vi "main_control_combo_F.vi"(6 "read":bool=TRUE) -> (9 "chiller readout":string, 10 "bytes read":u32)   [LabVIEW 2019]
doc: "The Basic Serial Read and Write example performs a Serial Port Read, a Serial Port Write, or a combination of these actions. The user selects the actions (read or write) on the front panel. If both are selected, the VI will write the data first, read data, and then close the VISA session that is opened to the port. This VI will wait until the specified number of bytes is received at the port. Only the number of bytes specified will be read.\n\nINSTRUCTIONS:\n1) Select the serial resource and configuration parameters (baud rate, data bits, parity, stop bits, flow control).\n2) Select the operations to be performed. \n3) Connect the serial port to your device. If no device is available, perform a loopback test by doing one of the following. Short pins 2 and 3 on a RS-232 cable or short pin 4 to pin 8 and pin 5 to pin 9 on a RS-485/422 cable. \n4) Run the VI to see the data read. (The \"read string\" will match the \"string to write\" if a loopback test was performed.)\n\nNote: The parameters set for the serial port must match the parameters of the connected instrument or device. In this example, the bytes to read parameter specifies the number of bytes that the serial port reads. If there were more bytes at the port than the number specified in bytes to read, those bytes would not be read. Also, if you specify to read more bytes than the number of bytes actually read, you might receive a timeout error message.\n\nOn the block diagram, the Configure Serial Port VI sets the configuration parameters. The front panel displays the controls used to configure the basic parameters, such as baud rate, data bits, and parity. Constants configure the other parameters the user probably does not need set. After the VISA Configure Serial Port VI opens the VISA session and configures the port, the VI passes the VISA resource name to other VIs that perform operations on that VISA resource. The VISA Write function sends a command to the serial device and the VISA Read function returns data based on the command. The VISA Close function then closes the reference to the serial device. It is important to close the reference; otherwise communication through with that port through protocols other than VISA might not be possible."
uses:
  <vilib>/Instr/_visa.llb/VISA Configure Serial Port (Instr).vi
  <vilib>/Utility/file.llb/Read Delimited Spreadsheet (string).vi
  Keithley/Keithley 24XX/Public/Data/Read (Single Point).vi
  Keithley/Keithley 24XX/Keithley 24XX.lvlib
  DELTA ELEKTRONIKA SM Series/DELTA ELEKTRONIKA.lvlib
  <resource>/objmgr/ni.var.rc
panel:
  out "specific error cleared?":bool
  out "manualDelta":bool
  out "read string 7":string
  out "delta readout":string
  in  "delay before read (ms) 4":u32=500
  in  "Combo Box 4":string(combo)
  in  "voltage delta":dbl
  out "delta command":string
  in  "write 4":bool
  in  "stop reading script":bool
  out "bytes read 6":u32
  out "read string 6":string
  out "concatenated string":string
  out "dewpoint":string
  out "temperature":string
  out "humidity":string
  out "n2 flow temperature":string
  out "dewpoint":string
  out "Current Limit 2":bool
  out "Voltage Limit 2":bool
  out "bytes read 5":u32
  out "read string 5":string
  out "bytes read 4":u32
  out "read string 4":string
  out "From Linux Box":string
  in  "Voltage Manual Range (1.0) 2":dbl=1.0
  in  "Current Manual Range (1.0) 2":dbl=1.0
  in  "Resistance Manual Range (1.0) 2":dbl=1.0
  in  "Enable Voltage Auto Range (T:Enable) 2":bool=TRUE
  in  "Enable Current Auto Range (T:Enable) 2":bool=TRUE
  in  "Enable Resistance Auto Range (T:Enable) 2":bool=TRUE
  out "Voltage 3":sgl
  out "Current 3":sgl
  out "Resistance 2":sgl
  out "Current Micro 2":sgl
  out "Command Log and Output":string
  out "COMBO COMMAND":string
  out "all rows":string[][](array[string])
  out "element":i32
  out "current command":string[](array[string])
  out "current argument":string[](array[string])
  out "size(s)":i32
  in  "file path (dialog if empty) 2":path
  in  "Read Script":bool
  in  "Enable Resistance Auto Range (T:Enable)":bool=TRUE
  out "relay TTi":errorcluster
  out "bytes read 3":u32
  out "inverter readout":string
  in  "read 3":bool=TRUE
  in  "delay before read (ms) 3":u32=500
  in  "Combo Box 3":string(combo)="VO?\n"
  in  "voltage or current 2":dbl
  out "string from combo 3":string
  in  "write 3":bool
  out "LV TTi":errorcluster
  out "bytes read 2":u32
  out "LVPS reaout":string
  in  "read 2":bool=TRUE
  in  "delay before read (ms) 2":u32=500
  in  "Combo Box 2":string(combo)="VO?\n"
  in  "voltage or current":dbl
  in  "write 2":bool
  in  "write":bool
  out "string from combo":string
  in  "Temperature":dbl
  in  "Combo Box":string(combo)
  out "Chiller":errorcluster
  out "N2 temperature > dew point + 2C":bool
  in  "File Path of rotonic datalog":path
  out "time humidity temporature dewpoint":string[](array[string])
  in  "Quit":bool
  in  "delay before read (ms)":u32=500
  # "Kiethley Powersupply"
  # "µA"
  # "Delta powersupply Interface"
  # "TTi LV powersupply Interface\nCOM 5 is default"
  # "Medical Chiller Interface\nCOM 6 is default"
  # "TTi LV powersupply Interface for the relay polarity control\nCOM 4 is default"
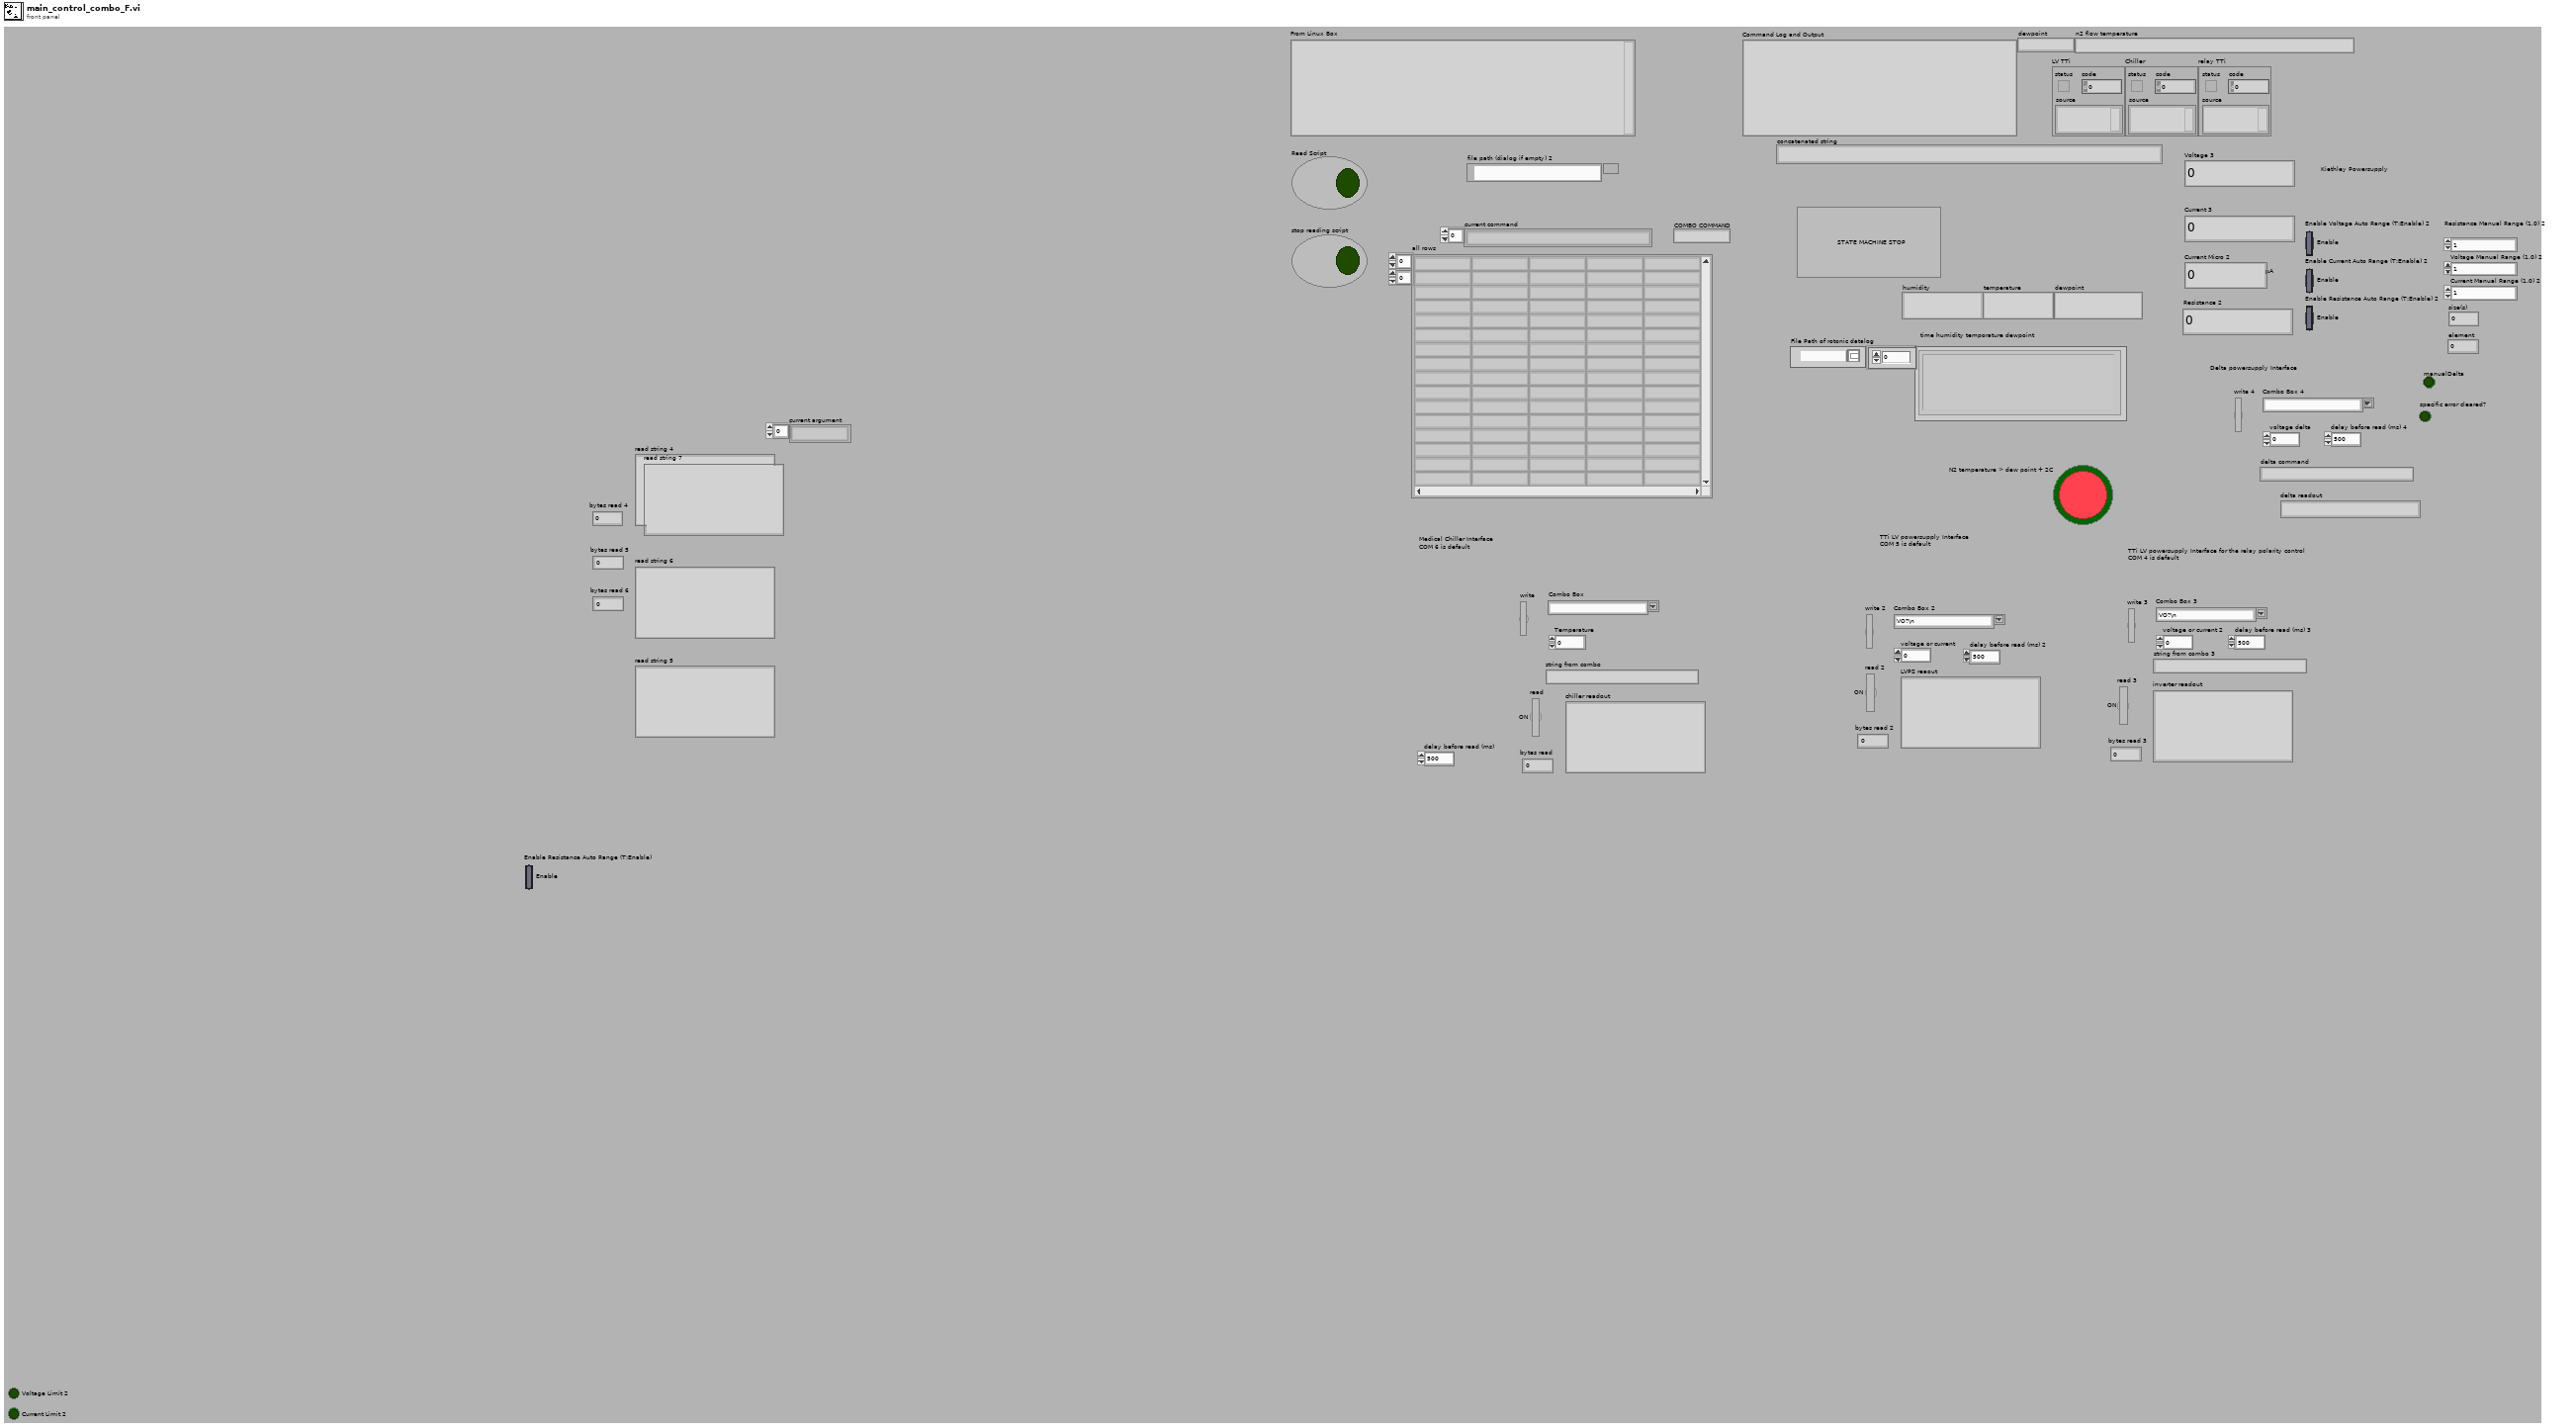
[diagram p1: front panel]
types:
  T1 = cluster{"Baud Rate":u32, "Parity":u16, "Data Bits":u16, "Stop Bits":u16, "Flow Control":u16}
  T2 = enum16{"open", "replace", "create", "open or create", "replace or create", "replace or create with confirmation"}
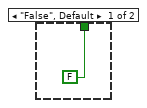
[diagram p2: hidden frame]
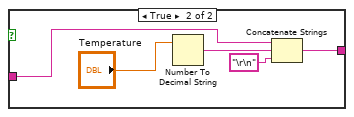
[diagram p4: hidden frame]
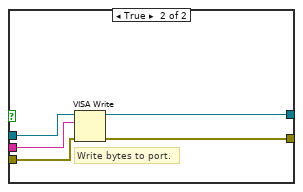
[diagram p5: hidden frame]
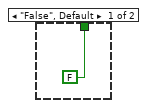
[diagram p7: hidden frame]
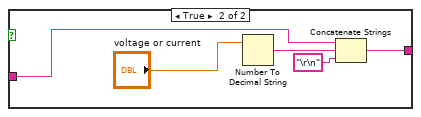
[diagram p9: hidden frame]
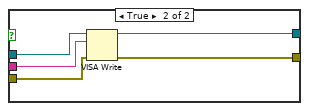
[diagram p10: hidden frame]
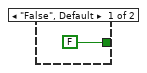
[diagram p12: hidden frame]
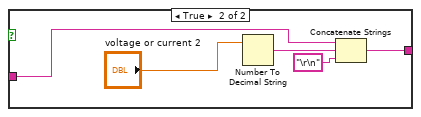
[diagram p14: hidden frame]
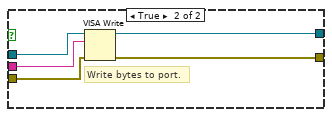
[diagram p15: hidden frame]
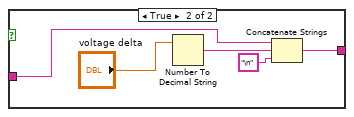
[diagram p18: hidden frame]
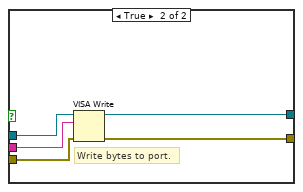
[diagram p19: hidden frame]
diagram:
  # "First save permanent values in non-volatile memory via NI - Max and the *SAV after setting it via SO:VO:MA 52 and SO:CU:MA 30    !"
  n1 = flat-sequence {
    tunnel: [w37] -> w11
    tunnel: [w36] -> w10
    tunnel: [w28] -> w8
    tunnel: [w27] -> w7
    tunnel: [w23] -> w6
    tunnel: [w22] -> w5
    tunnel: [w19] -> w4
    tunnel: [w18] -> w3
    tunnel: [w55] -> w17
    tunnel: [w54] -> w16
    tunnel: [w53] -> w15
    tunnel: [w52] -> w14
    tunnel: [w51] -> w13
    tunnel: w11 -> [w50]
    tunnel: w10 -> [w49]
    tunnel: [w48] -> w9
    tunnel: w8 -> [w47]
    tunnel: w7 -> [w46]
    tunnel: w6 -> [w45]
    tunnel: w5 -> [w44]
    tunnel: w4 -> [w43]
    tunnel: w3 -> [w42]
    tunnel: [w41] -> w2
    tunnel: [w40] -> w1
    tunnel: w17 -> [w661]
    tunnel: w16 -> [w659]
    tunnel: w15 -> [w658]
    tunnel: w14 -> [w656]
    tunnel: w13 -> [w655]
    tunnel: w9 -> [w654]
    tunnel: w2 -> [w653]
    tunnel: w1 -> [w652]
    frame #0 {
      w20 = u32 15000  # timeout (10sec)
      w24 = FALSE  # Enable Termination Char (T)
      w25 = u32 10000  # timeout (10sec)
      w29 = FALSE  # Enable Termination Char (T)
      w30 = u32 10000  # timeout (10sec)
      w35 = u32 10000  # timeout (10sec)
      w33 = FALSE  # Enable Termination Char (T)
      n2 = call "Initialize.vi"("Serial Configuration"=T1 {"Baud Rate"=9600, "Parity"=0, "Data Bits"=8, "Stop Bits"=10, "Flow Control"=1}, "Reset (True)"=FALSE, "VISA resource name"=refnum<visa-resource-name> "COM1" ("VISA resource name 4")) -> ()  [unwired: 7 in, 2 out]
      n3 = call-poly "VISA Configure Serial Port"("VISA resource name"=refnum<visa-resource-name> "COM4", "timeout (10sec)"=w35, "Enable Termination\nChar (T)"=w33) -> ("VISA resource name out"=w36:refnum<visa-resource-name>, "error out"=w37:errorcluster)  [unwired: 11 in]
      n4 = VISA Open(timeout (0)=w20, VISA resource name=refnum<visa-resource-name> "GPIB0::8::INSTR") -> (VISA resource name=w19:refnum<visa-resource-name>, error out=w18:errorcluster)  [unwired: 3 in]
      n5 = call-poly "VISA Configure Serial Port"("VISA resource name"=refnum<visa-resource-name> "COM5", "timeout (10sec)"=w25, "Enable Termination\nChar (T)"=w24) -> ("VISA resource name out"=w22:refnum<visa-resource-name>, "error out"=w23:errorcluster)  [unwired: 11 in]
      n6 = call-poly "VISA Configure Serial Port"("VISA resource name"=refnum<visa-resource-name> "COM6", "timeout (10sec)"=w30, "Enable Termination\nChar (T)"=w29) -> ("VISA resource name out"=w28:refnum<visa-resource-name>, "error out"=w27:errorcluster)  [unwired: 11 in]
    }
    frame #1 {
      # "Disable Output"
      # "State machine for iterating through commands from table"
      n7 = while {
        tunnel: ["Quit"] -> _
        stop <- "Quit" stop-if-true
      }
      n8 = while {
        stop <- w367 stop-if-true
        n9 = local read "Quit"() -> (w367:bool)
        n10 = case shown="True" "Read Script" {
          frame False {
          }
          frame True {
            n11 = Get Date/Time String() -> (date string=w391:string, time string=w389:string)  [unwired: 3 in]
            n12 = Search and Replace String(replace all?=TRUE ("replace all? (F)"), input string=w391, search string="/", replace string="_" ("replace string (\"\")")) -> (result string=w390:string)  [unwired: 4 in, 3 out]
            n13 = Search and Replace String(input string=w389, search string=":", replace string="" ("replace string (\"\")")) -> (result string=w388:string)  [unwired: 5 in, 3 out]
            n14 = Concatenate Strings("C:\\Users\\CMSOTDSF.CERN\\ExecutedCommands\\" ("string"), "command_log_" ("string"), w390, "_" ("string"), w388, ".txt" ("string")) -> (w387:string)
            n15 = String To Path(string=w387) -> (path=w377:path)
            n16 = Open/Create/Replace File(file path (use dialog)=w377, operation (0:open)=T2."replace or create") -> (refnum out=w376:refnum<file>)  [unwired: 4 in, 2 out]
            n17 = Concatenate Strings("Command Log Header for Executed CSV commands " ("text"), "\r\n") -> (w369:string)
            n18 = Set File Position(offset (in bytes) (0)=i64 0, refnum=w376, from (0:start)=enum16{"start", "end", "current"}."end") -> (refnum out=w373:refnum<file>)  [unwired: 1 in, 1 out]
            n19 = Write to Text File(file (use dialog)=w373, text=w369) -> ()  [unwired: 2 in, 3 out]
            n20 = flat-sequence {
              tunnel: ["file path (dialog if empty) 2"] -> w394
              tunnel: [w397] -> w393
              tunnel: [w395] -> w392
              tunnel: w377 -> [w395]
              tunnel: w394 -> [_]
              tunnel: w393 -> [w400]
              tunnel: w392 -> [w399]
              frame #0 {
                # "read table from CSV"
                n21 = call-poly <vilib>:"Read Delimited Spreadsheet.vi"("file path (dialog if empty)"="file path (dialog if empty) 2", "delimiter (\\t)"="," ("delimiter (\\t)")) -> ("all rows"=w397:string[][])  [unwired: 8 in, 5 out]
              }
              frame #1 {
                n22 = Array Size(array=w400) -> (size(s)=w403:i32[])
                n23 = Index Array(array=w403, index #1=0 ("index"), index #2=1 ("index")) -> (element #1=w404:i32)  [unwired: 1 out]
                "element" <- w404
                n24 = for {
                  N: w404 -> [_]
                  tunnel: w400 -> [w421] mode=indexing
                  tunnel: w399 -> [w408]
                  stop <- w414 stop-if-true
                  n25 = local read "Quit"() -> (w416:bool)
                  n26 = Array Subset(array=w421) -> (w417:string[])  [unwired: 2 in]
                  "current command" <- w417
                  n27 = Or(x=w416, y="stop reading script") -> (x .or. y?=w414:bool)
                  n28 = Array Size(array=w417) -> (size(s)=w420:i32)
                  "size(s)" <- w420
                  n29 = Index Array(array=w417, index=0) -> (element=w418:string)
                  "COMBO COMMAND" <- w418
                  n30 = for {
                    N: w420 -> [_]
                    tunnel: w417 -> [w607]
                    i -> [w604]
                    n31 = Add(x=w604, y=1) -> (x+y=w603:i32)
                    n32 = Wait Until Next ms Multiple(millisecond multiple=u32 1000) -> ()  [unwired: 1 out]
                    n33 = Array Subset(array=w607, index=w603) -> (→"current argument":string[])  [unwired: 1 in]
                  }
                  n34 = case shown="\"setChiller\"" w418 {
                    tunnel: w417 -> [w429 w443 w468 w489 w512 w536 _ w550 w571 _]
                    tunnel: [w422 w440 w466 w486 w510 w532 _ _ _ w577] -> w407
                    frame "wait", Default {
                      n35 = Array Subset(array=w429, index=1) -> (w427:string[])  [unwired: 1 in]
                      n36 = Index Array(array=w427, index=0) -> (element=w423:string)
                      n37 = Decimal String To Number(string=w423) -> (number=w425:i32)  [unwired: 2 in, 1 out]
                      n38 = Wait (ms)(milliseconds to wait=w425) -> ()  [unwired: 1 out]
                      n39 = Concatenate Strings("Wait for ", w423) -> (w422:string)
                    }
                    frame "setLVPS" {
                      # "Read the number of bytes specified."
                      # "Write bytes to port."
                      # "MUST specify codes display with single \"\\\""
                      # "Configure Serial port (baud rate,\ndata bits, parity, stop bits and flow control)."
                      n40 = Array Subset(array=w443, index=1) -> (w448:string[])  [unwired: 1 in]
                      n41 = Index Array(array=w448, index #1=0 ("index"), index #2=1 ("index")) -> (element #1=w445:string)  [unwired: 1 out]
                      n42 = Decimal String To Number(string=w445) -> (number=w442:i32)  [unwired: 2 in, 1 out]
                      n43 = To Double Precision Float(number=w442) -> (double precision float=w439:dbl)
                      n44 = case shown="1" w439 {
                        tunnel: ["OP 0\n" ("Combo Box 4") "OP 1\n" ("Combo Box 4")] -> w438
                        frame 0, Default {
                        }
                        frame 1 {
                        }
                      }
                      n45 = VISA Write(VISA resource name=refnum<visa-resource-name> "COM5", write buffer=w438) -> (VISA resource name out=w431:refnum<visa-resource-name>, error out=w430:errorcluster)  [unwired: 1 in, 1 out]
                      n46 = property class="Instr"(reference=w431, error in=w430) -> (reference out=w433:refnum<visa-resource-name>, error out=w434:errorcluster, "Serial Settings:Number of Bytes at Serial Port"=w435:u32)
                      "bytes read 4" <- w435
                      n47 = VISA Read(VISA resource name=w433, byte count=w435, error in (no error)=w434) -> (read buffer=w436:string, error out=w432:errorcluster)  [unwired: 2 out]
                      "read string 4" <- w436
                      n48 = Concatenate Strings("we just set the LV PS voltage to ", w436) -> (w440:string)
                      n49 = call <vilib>:"Simple Error Handler.vi"("error in (no error)"=w432) -> ()  [unwired: 4 in, 5 out]
                    }
                    frame "setDeltaPS" {
                      # "MUST specify codes display with single \"\\\""
                      # "Configure Serial port (baud rate,\ndata bits, parity, stop bits and flow control)."
                      n50 = Array Subset(array=w468, index=1) -> (w472:string[])  [unwired: 1 in]
                      n51 = Index Array(array=w472, index #1=0 ("index"), index #2=1 ("index")) -> (element #1=w459:string)  [unwired: 1 out]
                      n52 = Concatenate Strings("SOUR:VO " ("format string"), w459, "\n" ("string")) -> (w460:string)
                      n53 = VISA Write(VISA resource name=refnum<visa-resource-name> "GPIB0::8::INSTR", write buffer=w460) -> (VISA resource name out=w457:refnum<visa-resource-name>, error out=w456:errorcluster)  [unwired: 1 in, 1 out]
                      n54 = stacked-sequence {
                        tunnel: w456 -> [w475]
                        tunnel: [w475] -> w455
                        tunnel: w457 -> [w474]
                        tunnel: [w474] -> w453
                        frame #0 {
                          n55 = Wait (ms)(milliseconds to wait=u32 500) -> ()  [unwired: 1 out]
                        }
                      }
                      n56 = VISA Write(VISA resource name=w453, write buffer="ME:VO?\n", error in (no error)=w455) -> (VISA resource name out=w451:refnum<visa-resource-name>, error out=w454:errorcluster)  [unwired: 1 out]
                      n57 = VISA Read(VISA resource name=w451, byte count=u32 1024, error in (no error)=w454) -> (read buffer=w464:string, error out=w463:errorcluster)  [unwired: 2 out]
                      "read string 7" <- w464
                      n58 = Concatenate Strings("we just set the Delta voltage to ", w464) -> (w466:string)
                      n59 = call <vilib>:"Simple Error Handler.vi"("error in (no error)"=w463) -> ()  [unwired: 4 in, 5 out]
                    }
                    frame "setInverter" {
                      # "Read the number of bytes specified."
                      # "Write bytes to port."
                      # "MUST specify codes display with single \"\\\""
                      # "Configure Serial port (baud rate,\ndata bits, parity, stop bits and flow control)."
                      n60 = Array Subset(array=w489, index=1) -> (w494:string[])  [unwired: 1 in]
                      n61 = Index Array(array=w494, index #1=0 ("index"), index #2=1 ("index")) -> (element #1=w491:string)  [unwired: 1 out]
                      n62 = Decimal String To Number(string=w491) -> (number=w488:i32)  [unwired: 2 in, 1 out]
                      n63 = To Double Precision Float(number=w488) -> (double precision float=w485:dbl)
                      n64 = case shown="0, Default" w485 {
                        tunnel: ["OP 0\n" ("Combo Box 4") "OP 1\n" ("Combo Box 4")] -> w484
                        frame 0, Default {
                        }
                        frame 1 {
                        }
                      }
                      n65 = VISA Write(VISA resource name=refnum<visa-resource-name> "COM4", write buffer=w484) -> (VISA resource name out=w477:refnum<visa-resource-name>, error out=w476:errorcluster)  [unwired: 1 in, 1 out]
                      n66 = property class="Instr"(reference=w477, error in=w476) -> (reference out=w479:refnum<visa-resource-name>, error out=w480:errorcluster, "Serial Settings:Number of Bytes at Serial Port"=w481:u32)
                      "bytes read 6" <- w481
                      n67 = VISA Read(VISA resource name=w479, byte count=w481, error in (no error)=w480) -> (read buffer=w482:string, error out=w478:errorcluster)  [unwired: 2 out]
                      "read string 6" <- w482
                      n68 = Concatenate Strings("we just set the Inverter voltage to ", w482) -> (w486:string)
                      n69 = call <vilib>:"Simple Error Handler.vi"("error in (no error)"=w478) -> ()  [unwired: 4 in, 5 out]
                    }
                    frame "setChiller" {
                      # "Read the number of bytes specified."
                      # "Write bytes to port."
                      # "MUST specify codes display with single \"\\\""
                      # "Configure Serial port (baud rate,\ndata bits, parity, stop bits and flow control)."
                      n70 = Array Subset(array=w512, index=1) -> (w516:string[])  [unwired: 1 in]
                      n71 = Index Array(array=w516, index #1=0 ("index"), index #2=1 ("index")) -> (element #1=w498:string, element #2=w500:string)
                      n72 = Decimal String To Number(string=w500) -> (number=w499:i32)  [unwired: 2 in, 1 out]
                      n73 = To Double Precision Float(number=w499) -> (double precision float=w497:dbl)
                      n74 = case shown="\"settemp\"" w498 {
                        tunnel: ["STOP\n" ("Combo Box 4") "START\n" ("Combo Box 4") w520] -> w509
                        tunnel: w497 -> [_ _ w519]
                        frame "stop", Default {
                        }
                        frame "start" {
                        }
                        frame "settemp" {
                          n75 = Number To Decimal String(number=w519) -> (decimal integer string=w523:string)  [unwired: 1 in]
                          n76 = Concatenate Strings("OUT_SP_00_" ("Combo Box 4"), w523, "\r\n" ("string")) -> (w520:string)
                        }
                      }
                      n77 = VISA Write(VISA resource name=refnum<visa-resource-name> "COM6", write buffer=w509) -> (VISA resource name out=w502:refnum<visa-resource-name>, error out=w501:errorcluster)  [unwired: 1 in, 1 out]
                      n78 = property class="Instr"(reference=w502, error in=w501) -> (reference out=w504:refnum<visa-resource-name>, error out=w505:errorcluster, "Serial Settings:Number of Bytes at Serial Port"=w506:u32)
                      "bytes read 5" <- w506
                      n79 = VISA Read(VISA resource name=w504, byte count=w506, error in (no error)=w505) -> (read buffer=w507:string, error out=w503:errorcluster)  [unwired: 2 out]
                      "read string 5" <- w507
                      n80 = Concatenate Strings("we just set the Chiller temperature to ", w507) -> (w510:string)
                      n81 = call <vilib>:"Simple Error Handler.vi"("error in (no error)"=w503) -> ()  [unwired: 4 in, 5 out]
                    }
                    frame "keithleynew" {
                      w524 = u16 0 items=["Voltage", "Current"] ("Source Mode  (0: Voltage)")
                      # "Configure each of the three measurements. settings"
                      n82 = Array Subset(array=w536, index=1) -> (w539:string[])  [unwired: 1 in]
                      n83 = Index Array(array=w539, index #1=0 ("index"), index #2=1 ("index")) -> (element #1=w533:string)  [unwired: 1 out]
                      n84 = Decimal String To Number(string=w533) -> (number=w535:i32)  [unwired: 2 in, 1 out]
                      n85 = To Double Precision Float(number=w535) -> (double precision float=w530:dbl)
                      n86 = Concatenate Strings("we just set the keithley voltage to ", w533) -> (w532:string)
                      n87 = call "Configure Output.vi"("Source Mode  (0: Voltage)"=w524, "Compliance  Level (0.1)"=1e-05, "Output Level (0)"=w530, "VISA resource name"=refnum<visa-resource-name> "COM1") -> ("error out"=w528:errorcluster, "VISA resource name out"=w529:refnum<visa-resource-name>)  [unwired: 6 in]
                      n88 = call "Enable Output.vi"("error in (no error)"=w528, "Enable Output (T: Enable)"=TRUE, "VISA resource name"=w529) -> ()  [unwired: 7 in, 2 out]
                    }
                    frame "closekeithley" {
                      n89 = call "Enable Output.vi"("Enable Output (T: Enable)"=FALSE, "VISA resource name"=refnum<visa-resource-name> "COM1") -> ("error out"=w541:errorcluster, "VISA resource name out"=w542:refnum<visa-resource-name>)  [unwired: 8 in]
                      n90 = call "Close.vi"("error in (no error)"=w541, "VISA resource name"=w542) -> ("error out"=w544:errorcluster)  [unwired: 9 in]
                      n91 = call <vilib>:"Simple Error Handler.vi"("error in (no error)"=w544) -> ()  [unwired: 4 in, 5 out]
                    }
                    frame "OldsetDeltaPS" {
                      w565 = TRUE  # Enable Output (T: Enable)
                      # "Read OVP and OCP Status and\nactual voltage and current levels"
                      # "Configure Output"
                      n92 = Array Subset(array=w550, index=1) -> (w555:string[])  [unwired: 1 in]
                      n93 = Index Array(array=w555, index #1=0 ("index"), index #2=1 ("index")) -> (element #1=w552:string, element #2=w547:string)
                      n94 = Decimal String To Number(string=w552) -> (number=w549:i32)  [unwired: 2 in, 1 out]
                      n95 = Decimal String To Number(string=w547) -> (number=w548:i32)  [unwired: 2 in, 1 out]
                      n96 = To Double Precision Float(number=w549) -> (double precision float=w545:dbl)
                      n97 = To Double Precision Float(number=w548) -> (double precision float=w546:dbl)
                      n98 = call "Configure Output Voltage.vi"("Set Voltage(0.0 V)"=w545, "VISA resource name"=refnum<visa-resource-name> "LPT1") -> ("error out"=w564:errorcluster, "VISA resource name out"=w563:refnum<visa-resource-name>)  [unwired: 8 in]
                      n99 = call "Configure Current Limit.vi"("error in (no error)"=w564, "Current Limit (0.0 A)"=w546, "VISA resource name"=w563) -> ("error out"=w566:errorcluster, "VISA resource name out"=w567:refnum<visa-resource-name>)  [unwired: 7 in]
                      n100 = call "Configure Output.vi"("Enable Output (T: Enable)"=w565, "error in (no error)"=w566, "VISA resource name"=w567) -> ("error out"=w557:errorcluster, "VISA resource name out"=w556:refnum<visa-resource-name>)  [unwired: 7 in]
                      n101 = call "Output Protection Status.vi"("error in (no error)"=w557, "VISA resource name"=w556) -> ("error out"=w559:errorcluster, "OCP Tripped?"=→"Current Limit 2":bool, "OVP Tripped?"=→"Voltage Limit 2":bool, "VISA resource name out"=w558:refnum<visa-resource-name>)  [unwired: 6 in]
                      n102 = call "Read Output.vi"("error in (no error)"=w559, "VISA resource name"=w558) -> ()  [unwired: 6 in, 4 out]
                    }
                    frame "dumsetDeltaPS" {
                      n103 = Array Subset(array=w571, index=1) -> (w576:string[])  [unwired: 1 in]
                      n104 = Index Array(array=w576, index #1=0 ("index"), index #2=1 ("index")) -> (element #1=w573:string, element #2=w568:string)
                      n105 = Decimal String To Number(string=w573) -> (number=w570:i32)  [unwired: 2 in, 1 out]
                      n106 = Decimal String To Number(string=w568) -> (number=w569:i32)  [unwired: 2 in, 1 out]
                      n107 = To Double Precision Float(number=w570) -> ()  [unwired: 1 out]
                      n108 = To Double Precision Float(number=w569) -> ()  [unwired: 1 out]
                    }
                    frame "2sCalibration" {
                      # "C:\\Users\\CMSOTDSF.CERN\\2sCalibrationOut"
                      # "run a windows batch file that will call ssh command with an INPUT bash script\nThe input bash script will run the 2s calibration and is located here:\nC:\\Users\\CMSOTDSF.CERN\\cc7.sh"
                      n109 = flat-sequence {
                        tunnel: [w580] -> w578
                        tunnel: w578 -> [w586]
                        tunnel: [w585] -> w577
                        frame #0 {
                          n110 = call <vilib>:"System Exec.vi"("run minimized? (F)"=TRUE, "working directory"=path "C:/Users/CMSOTDSF.CERN/OpenSSH", "command line"="cmd /c C:\\Users\\CMSOTDSF.CERN\\windows_cc7.bat") -> ("standard error"=w581:string, "standard output"=w582:string)  [unwired: 5 in, 2 out]
                          "From Linux Box" <- w582
                          n111 = Concatenate Strings(w582, w581) -> (w580:string)
                        }
                        frame #1 {
                          n112 = Get Date/Time String() -> (date string=w597:string, time string=w599:string)  [unwired: 3 in]
                          n113 = Search and Replace String(input string=w599, search string=":", replace string="" ("replace string (\"\")")) -> (result string=w600:string)  [unwired: 5 in, 3 out]
                          n114 = Search and Replace String(replace all?=TRUE ("replace all? (F)"), input string=w597, search string="/", replace string="_" ("replace string (\"\")")) -> (result string=w598:string)  [unwired: 4 in, 3 out]
                          n115 = Concatenate Strings("C:\\Users\\CMSOTDSF.CERN\\2sCalibrationOut\\" ("string"), "2scalibration_" ("string"), w598, "_" ("string"), w600, ".txt" ("string")) -> (w601:string)
                          n116 = String To Path(string=w601) -> (path=w602:path)
                          n117 = Concatenate Strings("2S Calibration done output is saved to: ", w601) -> (w585:string)
                          n118 = Write to Text File(file (use dialog)=w602, text=w586) -> ()  [unwired: 2 in, 3 out]
                        }
                      }
                    }
                  }
                  "Command Log and Output" <- w407
                  n119 = Open/Create/Replace File(file path (use dialog)=w408, operation (0:open)=T2."open") -> (refnum out=w409:refnum<file>)  [unwired: 4 in, 2 out]
                  n120 = Concatenate Strings(w407, "\r\n") -> (w406:string)
                  n121 = Set File Position(offset (in bytes) (0)=i64 0, refnum=w409, from (0:start)=enum16{"start", "end", "current"}."end") -> (refnum out=w411:refnum<file>)  [unwired: 1 in, 1 out]
                  n122 = Write to Text File(file (use dialog)=w411, text=w406) -> ()  [unwired: 2 in, 3 out]
                }
                "all rows" <- w400
              }
              frame #2 {
                n123 = invoke on="Read Script" class="Bool (strict)" method="Reinit To Default"() -> ()  [unwired: 3 in, 3 out]
                n124 = local write "COMBO COMMAND"("" ("COMBO COMMAND")) -> ()
              }
            }
          }
        }
      }
      n125 = while {
        tunnel: w43 -> [w266]
        tunnel: [w260] -> w41
        tunnel: w42 -> [w265]
        tunnel: [w259] -> w40
        stop <- w261 stop-if-true
        n126 = local read "COMBO COMMAND"() -> (w256:string)
        n127 = Search and Replace String(input string=w256, search string="setDeltaPS", replace string="True" ("replace string (\"\")")) -> (result string=w262:string)  [unwired: 5 in, 3 out]
        n128 = case shown="\"False\", Default" w262 {
          tunnel: [FALSE TRUE] -> w263
          frame "False", Default {
          }
          frame "True" {
          }
        }
        n129 = local read "Quit"() -> (w264:bool)
        n130 = Or(x=w263, y=w264) -> (x .or. y?=w258:bool)
        n131 = Not(x=w258) -> (.not. x?=w257:bool)
        "manualDelta" <- w257
        n132 = case shown="True" w257 {
          tunnel: w266 -> [w268 w272]
          tunnel: w265 -> [w267 w271]
          tunnel: [w268 w270] -> w260
          tunnel: [w267 w269] -> w259
          frame False {
          }
          frame True {
            n133 = while {
              tunnel: w272 -> [w292]
              tunnel: [w278] -> w270
              tunnel: w271 -> [w275]
              tunnel: [w277] -> w269
              stop <- FALSE stop-if-true
              # "delta"
              # "Configure Serial port (baud rate,\ndata bits, parity, stop bits and flow control)."
              n134 = call <vilib>:"Clear Errors.vi"("error in (no error)"=w275, "specific error code to clear (0: all)"=-1073807339.0 ("y")) -> ("error out"=w274:errorcluster, "specific error cleared?"=→"specific error cleared?":bool)  [unwired: 4 in]
              n135 = Match True/False String(2:"" ("false string"), 3:"SOUR:VO " ("format string"), 4:"Combo Box 4") -> (0:w285:bool)  [unwired: 1 out]
              n136 = case shown="False" w285 {
                tunnel: [w293 w296] -> w282
                tunnel: "Combo Box 4" -> [w293 w295]
                frame False {
                }
                frame True {
                  n137 = Number To Decimal String(number="voltage delta") -> (decimal integer string=w298:string)  [unwired: 1 in]
                  n138 = Concatenate Strings(w295, w298, "\n" ("string")) -> (w296:string)
                }
              }
              "delta command" <- w282
              n139 = case shown="False" "write 4" {
                tunnel: [w302 w311] -> w291
                tunnel: w292 -> [w306 w310]
                tunnel: w274 -> [w305 w309]
                tunnel: [w303 w308] -> w289
                tunnel: w282 -> [_ w307]
                frame False {
                  n140 = VISA Write(VISA resource name=w306, write buffer="ME:VO?\n", error in (no error)=w305) -> (VISA resource name out=w303:refnum<visa-resource-name>, error out=w302:errorcluster)  [unwired: 1 out]
                }
                frame True {
                  # "Write bytes to port."
                  n141 = VISA Write(VISA resource name=w310, write buffer=w307, error in (no error)=w309) -> (VISA resource name out=w308:refnum<visa-resource-name>, error out=w311:errorcluster)  [unwired: 1 out]
                }
              }
              n142 = stacked-sequence {
                tunnel: w291 -> [w301]
                tunnel: [w301] -> w290
                tunnel: w289 -> [w300]
                tunnel: [w300] -> w288
                frame #0 {
                  n143 = Wait (ms)(milliseconds to wait="delay before read (ms) 4") -> ()  [unwired: 1 out]
                }
              }
              n144 = Not(x="write 4") -> (.not. x?=w280:bool)
              n145 = case shown="True" w280 {
                tunnel: w290 -> [w313 w314]
                tunnel: [w313 w319] -> w277
                tunnel: [w312 w318] -> w278
                tunnel: w288 -> [w312 w316]
                frame False {
                }
                frame True {
                  # "Read the number of bytes specified."
                  n146 = VISA Read(VISA resource name=w316, byte count=u32 1024, error in (no error)=w314) -> (VISA resource name out=w318:refnum<visa-resource-name>, read buffer=→"delta readout":string, error out=w319:errorcluster)  [unwired: 1 out]
                }
              }
              n147 = Wait Until Next ms Multiple(millisecond multiple=u32 50) -> ()  [unwired: 1 out]
            }
          }
        }
        n148 = local read "Quit"() -> (w261:bool)
      }
      n149 = while {
        tunnel: w44 -> [w132]
        tunnel: [w134] -> w51
        tunnel: w45 -> [w133]
        tunnel: [w135] -> w52
        stop <- w131 stop-if-true
        n150 = local read "COMBO COMMAND"() -> (w127:string)
        n151 = Search and Replace String(input string=w127, search string="setLVPS", replace string="True" ("replace string (\"\")")) -> (result string=w128:string)  [unwired: 5 in, 3 out]
        n152 = case shown="\"True\"" w128 {
          tunnel: [FALSE TRUE] -> w129
          frame "False", Default {
          }
          frame "True" {
          }
        }
        n153 = local read "Quit"() -> (w130:bool)
        n154 = Or(x=w129, y=w130) -> (x .or. y?=w124:bool)
        n155 = Not(x=w124) -> (.not. x?=w123:bool)
        n156 = case shown="True" w123 {
          tunnel: [w138 w143] -> w135
          tunnel: [w139 w142] -> w134
          tunnel: w133 -> [w138 w141]
          tunnel: w132 -> [w139 w140]
          frame False {
          }
          frame True {
            n157 = while {
              shift-right: [w157] -> w143
              shift-left: w141 -> [w159]
              shift-right: [w156] -> w142
              shift-left: w140 -> [w158]
              stop <- FALSE stop-if-true
              # "TTi SEH PS LV"
              n158 = Match True/False String(2:"" ("false string"), 3:"OUT_SP_00_" ("format string"), 4:"Combo Box 2") -> (0:w149:bool)  [unwired: 1 out]
              n159 = case shown="False" w149 {
                tunnel: [w161 w164] -> w146
                tunnel: "Combo Box 2" -> [w161 w163]
                frame False {
                }
                frame True {
                  n160 = Number To Decimal String(number="voltage or current") -> (decimal integer string=w166:string)  [unwired: 1 in]
                  n161 = Concatenate Strings(w163, w166, "\r\n" ("string")) -> (w164:string)
                }
              }
              n162 = case shown="False" "write 2" {
                tunnel: [w171 w176] -> w155
                tunnel: w158 -> [w170 w175]
                tunnel: w159 -> [w171 w174]
                tunnel: [w170 w173] -> w153
                tunnel: w146 -> [_ w172]
                frame False {
                }
                frame True {
                  n163 = VISA Write(VISA resource name=w175, write buffer=w172, error in (no error)=w174) -> (VISA resource name out=w173:refnum<visa-resource-name>, error out=w176:errorcluster)  [unwired: 1 out]
                }
              }
              n164 = stacked-sequence {
                tunnel: w155 -> [w169]
                tunnel: [w169] -> w154
                tunnel: w153 -> [w168]
                tunnel: [w168] -> w152
                frame #0 {
                  n165 = Wait (ms)(milliseconds to wait="delay before read (ms) 2") -> ()  [unwired: 1 out]
                }
              }
              n166 = case shown="True" "read 2" {
                tunnel: w154 -> [w178 w182]
                tunnel: [w178 w186] -> w157
                tunnel: [w177 w185] -> w156
                tunnel: w152 -> [w177 w184]
                frame False {
                }
                frame True {
                  # "Read the number of bytes specified."
                  n167 = property class="Instr"(reference=w184, error in=w182) -> (reference out=w183:refnum<visa-resource-name>, error out=w181:errorcluster, "Serial Settings:Number of Bytes at Serial Port"=w180:u32)
                  "bytes read 2" <- w180
                  n168 = VISA Read(VISA resource name=w183, byte count=w180, error in (no error)=w181) -> (VISA resource name out=w185:refnum<visa-resource-name>, read buffer=→"LVPS reaout":string, error out=w186:errorcluster)  [unwired: 1 out]
                }
              }
              n169 = Wait Until Next ms Multiple(millisecond multiple=u32 50) -> ()  [unwired: 1 out]
            }
          }
        }
        n170 = local read "Quit"() -> (w131:bool)
      }
      n171 = while {
        tunnel: w50 -> [w197]
        tunnel: [w199] -> w54
        tunnel: w49 -> [w196]
        tunnel: [w198] -> w53
        stop <- w195 stop-if-true
        n172 = local read "COMBO COMMAND"() -> (w194:string)
        n173 = Search and Replace String(input string=w194, search string="setInverter", replace string="True" ("replace string (\"\")")) -> (result string=w193:string)  [unwired: 5 in, 3 out]
        n174 = case shown="\"True\"" w193 {
          tunnel: [FALSE TRUE] -> w190
          frame "False", Default {
          }
          frame "True" {
          }
        }
        n175 = local read "Quit"() -> (w189:bool)
        n176 = Or(x=w190, y=w189) -> (x .or. y?=w188:bool)
        n177 = Not(x=w188) -> (.not. x?=w187:bool)
        n178 = case shown="True" w187 {
          tunnel: [w203 w207] -> w199
          tunnel: [w202 w206] -> w198
          tunnel: w197 -> [w203 w205]
          tunnel: w196 -> [w202 w204]
          frame False {
          }
          frame True {
            n179 = while {
              shift-right: [w222] -> w207
              shift-left: w205 -> [w223]
              shift-right: [w221] -> w206
              shift-left: w204 -> [w209]
              stop <- FALSE stop-if-true
              # "RELAY LV PS"
              # "Configure Serial port (baud rate,\ndata bits, parity, stop bits and flow control)."
              n180 = Match True/False String(2:"" ("false string"), 3:"OUT_SP_00_" ("format string"), 4:"Combo Box 3") -> (0:w214:bool)  [unwired: 1 out]
              n181 = case shown="False" w214 {
                tunnel: [w225 w228] -> w211
                tunnel: "Combo Box 3" -> [w225 w227]
                frame False {
                }
                frame True {
                  n182 = Number To Decimal String(number="voltage or current 2") -> (decimal integer string=w230:string)  [unwired: 1 in]
                  n183 = Concatenate Strings(w227, w230, "\r\n" ("string")) -> (w228:string)
                }
              }
              "string from combo 3" <- w211
              n184 = case shown="False" "write 3" {
                tunnel: [w235 w243] -> w220
                tunnel: w209 -> [w238 w242]
                tunnel: w223 -> [w234 w241]
                tunnel: [w236 w240] -> w218
                tunnel: w211 -> [_ w239]
                frame False {
                  n185 = VISA Write(VISA resource name=w238, write buffer="VO?\n", error in (no error)=w234) -> (VISA resource name out=w236:refnum<visa-resource-name>, error out=w235:errorcluster)  [unwired: 1 out]
                }
                frame True {
                  # "Write bytes to port."
                  n186 = VISA Write(VISA resource name=w242, write buffer=w239, error in (no error)=w241) -> (VISA resource name out=w240:refnum<visa-resource-name>, error out=w243:errorcluster)  [unwired: 1 out]
                }
              }
              n187 = stacked-sequence {
                tunnel: w220 -> [w233]
                tunnel: [w233] -> w219
                tunnel: w218 -> [w232]
                tunnel: [w232] -> w217
                frame #0 {
                  n188 = Wait (ms)(milliseconds to wait="delay before read (ms) 3") -> ()  [unwired: 1 out]
                }
              }
              n189 = case shown="True" "read 3" {
                tunnel: w219 -> [w245 w249]
                tunnel: [w245 w253] -> w222
                tunnel: [w244 w252] -> w221
                tunnel: w217 -> [w244 w251]
                frame False {
                }
                frame True {
                  # "Read the number of bytes specified."
                  n190 = property class="Instr"(reference=w251, error in=w249) -> (reference out=w250:refnum<visa-resource-name>, error out=w248:errorcluster, "Serial Settings:Number of Bytes at Serial Port"=w247:u32)
                  "bytes read 3" <- w247
                  n191 = VISA Read(VISA resource name=w250, byte count=w247, error in (no error)=w248) -> (VISA resource name out=w252:refnum<visa-resource-name>, read buffer=→"inverter readout":string, error out=w253:errorcluster)  [unwired: 1 out]
                }
              }
              n192 = Wait Until Next ms Multiple(millisecond multiple=u32 50) -> ()  [unwired: 1 out]
            }
          }
        }
        n193 = local read "Quit"() -> (w195:bool)
      }
      n194 = while {
        tunnel: w47 -> [w66]
        tunnel: [w67] -> w48
        tunnel: w46 -> [w65]
        tunnel: [w68] -> w55
        stop <- w64 stop-if-true
        n195 = local read "COMBO COMMAND"() -> (w62:string)
        n196 = Search and Replace String(input string=w62, search string="setChiller", replace string="True" ("replace string (\"\")")) -> (result string=w60:string)  [unwired: 5 in, 3 out]
        n197 = case shown="\"True\"" w60 {
          tunnel: [FALSE TRUE] -> w61
          frame "False", Default {
          }
          frame "True" {
          }
        }
        n198 = local read "Quit"() -> (w63:bool)
        n199 = Or(x=w61, y=w63) -> (x .or. y?=w57:bool)
        n200 = Not(x=w57) -> (.not. x?=w56:bool)
        n201 = case shown="True" w56 {
          tunnel: [w71 w76] -> w68
          tunnel: [w72 w75] -> w67
          tunnel: w66 -> [w72 w74]
          tunnel: w65 -> [w71 w73]
          frame False {
          }
          frame True {
            n202 = while {
              shift-right: [w90] -> w76
              shift-left: w73 -> [w92]
              shift-right: [w89] -> w75
              shift-left: w74 -> [w91]
              stop <- FALSE stop-if-true
              # "CHILLER"
              # "Configure Serial port (baud rate,\ndata bits, parity, stop bits and flow control)."
              n203 = Match True/False String(2:"" ("false string"), 3:"OUT_SP_00_" ("format string"), 4:"Combo Box") -> (0:w82:bool)  [unwired: 1 out]
              n204 = case shown="False" w82 {
                tunnel: [w94 w97] -> w79
                tunnel: "Combo Box" -> [w94 w96]
                frame False {
                }
                frame True {
                  n205 = Number To Decimal String(number="Temperature") -> (decimal integer string=w99:string)  [unwired: 1 in]
                  n206 = Concatenate Strings(w96, w99, "\r\n" ("string")) -> (w97:string)
                }
              }
              "string from combo" <- w79
              n207 = case shown="False" "write" {
                tunnel: [w103 w112] -> w88
                tunnel: w91 -> [w107 w111]
                tunnel: w92 -> [w106 w110]
                tunnel: [w104 w109] -> w86
                tunnel: w79 -> [_ w108]
                frame False {
                  n208 = VISA Write(VISA resource name=w107, write buffer="IN_PV_00\r\n", error in (no error)=w106) -> (VISA resource name out=w104:refnum<visa-resource-name>, error out=w103:errorcluster)  [unwired: 1 out]
                }
                frame True {
                  # "Write bytes to port."
                  n209 = VISA Write(VISA resource name=w111, write buffer=w108, error in (no error)=w110) -> (VISA resource name out=w109:refnum<visa-resource-name>, error out=w112:errorcluster)  [unwired: 1 out]
                }
              }
              n210 = stacked-sequence {
                tunnel: w88 -> [w102]
                tunnel: [w102] -> w87
                tunnel: w86 -> [w101]
                tunnel: [w101] -> w85
                frame #0 {
                  n211 = Wait (ms)(milliseconds to wait="delay before read (ms)") -> ()  [unwired: 1 out]
                }
              }
              n212 = case shown="True" "read" {
                tunnel: w87 -> [w114 w118]
                tunnel: [w114 w122] -> w90
                tunnel: [w113 w121] -> w89
                tunnel: w85 -> [w113 w120]
                frame False {
                }
                frame True {
                  # "Read the number of bytes specified."
                  n213 = property class="Instr"(reference=w120, error in=w118) -> (reference out=w119:refnum<visa-resource-name>, error out=w117:errorcluster, "Serial Settings:Number of Bytes at Serial Port"=w116:u32)
                  "bytes read" <- w116
                  n214 = VISA Read(VISA resource name=w119, byte count=w116, error in (no error)=w117) -> (VISA resource name out=w121:refnum<visa-resource-name>, read buffer=→"chiller readout":string, error out=w122:errorcluster)  [unwired: 1 out]
                }
              }
              n215 = Wait Until Next ms Multiple(millisecond multiple=u32 50) -> ()  [unwired: 1 out]
            }
          }
        }
        n216 = local read "Quit"() -> (w64:bool)
      }
      n217 = while {
        stop <- w610 stop-if-true
        (unwired) "humidity_202105"
        (unwired) path "C:/Users/fengwang.PCCMSTKUPDSF2/Desktop/RotronicUSBDriver/dataLog" ("file (use dialog)")
        # "dew point"
        # "N2 flow temperature"
        # "Convert text file string to array"
        # "Return the Number of lines."
        # "Extract only the size dimension we need"
        # "Get the size of the array"
        # "Read Text File, dialog box if none"
        n218 = local read "Quit"() -> (w610:bool)
        n219 = Get Date/Time In Seconds() -> (seconds since 1Jan1904=w616:timestamp)
        n220 = Format Date/Time String(time format string (%c)="%d_%m_%Y", seconds (now)=w616) -> (date/time string=w614:string)  [unwired: 1 in]
        n221 = Concatenate Strings("C:\\Users\\fengwang.PCCMSTKUPDSF2\\Desktop\\RotronicUSBDriver\\dataLog\\humidity_", w614) -> (→"concatenated string":string)
        n222 = Read from Text File(file (use dialog)="File Path of rotonic datalog") -> (text=w643:string)  [unwired: 1 in, 5 out]
        n223 = Spreadsheet String To Array(delimiter (Tab)="\r", format string="%d", spreadsheet string=w643) -> (array=w641:dbl[][])  [unwired: 1 out]
        n224 = Array Size(array=w641) -> (size(s)=w642:i32[])
        n225 = Index Array(array=w642) -> (element=w645:i32)  [unwired: 1 in]
        n226 = Read from Text File(file (use dialog)="File Path of rotonic datalog", count=w645) -> (text=w646:string[])  [unwired: 1 in, 4 out]
        n227 = Decrement(x=w645) -> (x-1=w644:i32)
        n228 = Array Subset(array=w646, index=w644) -> (w647:string[])  [unwired: 1 in]
        "time humidity temporature dewpoint" <- w647
        n229 = Get Date/Time In Seconds() -> (seconds since 1Jan1904=w639:timestamp)
        n230 = Array To Spreadsheet String(array=w647, 3:"%d/%m/%Y %H:%M:%S %4.12f %4.12f %4.12f" ("time format string (%c)")) -> (spreadsheet string=w618:string)  [unwired: 1 in]
        n231 = Format Date/Time String(time format string (%c)="%d/%m/%Y %H:%M:%S ", seconds (now)=w639) -> (date/time string=w640:string)  [unwired: 1 in]
        n232 = String Subset(string=w618, offset (0)=20, length (rest)=5 ("length (rest)")) -> (substring=→"humidity":string)
        n233 = Scan From String(format string=w640, input string=w618) -> (remaining string=w648:string)  [unwired: 4 in, 2 out]
        n234 = String Subset(string=w618, offset (0)=27, length (rest)=5 ("length (rest)")) -> (substring=→"temperature":string)
        n235 = String Subset(string=w618, offset (0)=34, length (rest)=6 ("length (rest)")) -> (substring=w611:string)
        "dewpoint" <- w611
        n236 = property class="Variable Object" props=["ClassId"](reference=w611) -> ()  [unwired: 1 in, 3 out]
        n237 = String Subset(string=w648, offset (0)=12, length (rest)=5 ("length (rest)")) -> (substring=w649:string)
        "dewpoint" <- w649
        n238 = Fract/Exp String To Number(string=w649) -> (number=w629:dbl)  [unwired: 3 in, 1 out]
        n239 = String Subset(string=w648, offset (0)=6, length (rest)=5 ("length (rest)")) -> (substring=w627:string)
        "n2 flow temperature" <- w627
        n240 = Fract/Exp String To Number(string=w627) -> (number=w650:dbl)  [unwired: 3 in, 1 out]
        n241 = Add(x=w629, y=2.0) -> (x+y=w628:dbl)
        n242 = Greater?(x=w650, y=w628) -> (0:→"N2 temperature > dew point + 2C":bool)
        n243 = call <vilib>:"Simple Error Handler.vi"() -> ()  [unwired: 5 in, 5 out]
      }
      n244 = while {
        stop <- w323 stop-if-true
        n245 = local read "file path (dialog if empty) 2"() -> (w324:path)
        n246 = Equal?(x=w324, y=path "") -> (x = y?=w328:bool)
        n247 = case shown="False" w328 {
          tunnel: [w330 path "C:/LabVIEW/OuterTrackerControl/example_commands.csv"] -> w329
          tunnel: w324 -> [w330 _]
          frame False {
          }
          frame True {
          }
        }
        n248 = local read "Quit"() -> (w323:bool)
        n249 = call-poly <vilib>:"Read Delimited Spreadsheet.vi"("file path (dialog if empty)"=w329, "delimiter (\\t)"="," ("delimiter (\\t)")) -> ("all rows"=w327:string[][])  [unwired: 8 in, 5 out]
        n250 = local write "all rows"(w327) -> ()
      }
      n251 = while {
        stop <- w334 stop-if-true
        w350 = u16 0 items=["Volts", "Current", "Resistance"]  # Function (0: Volts)
        w357 = u16 2 items=["Volts", "Current", "Resistance"]  # Function (0: Volts)
        w358 = u16 1 items=["Volts", "Current", "Resistance"]  # Function (0: Volts)
        # "Take the readings."
        # "Configure the output."
        # "Configure each of the three measurements. settings"
        n252 = call "Configure Measurement.vi"("Manual Range (1.0)"="Voltage Manual Range (1.0) 2", "Enable Auto Range (T:Enable)"="Enable Voltage Auto Range (T:Enable) 2", "Function (0: Volts)"=w350, "VISA resource name"=refnum<visa-resource-name> "COM1") -> ("error out"=w361:errorcluster, "VISA resource name out"=w362:refnum<visa-resource-name>)  [unwired: 6 in]
        n253 = call "Configure Measurement.vi"("Manual Range (1.0)"="Current Manual Range (1.0) 2", "error in (no error)"=w361, "Enable Auto Range (T:Enable)"="Enable Current Auto Range (T:Enable) 2", "Function (0: Volts)"=w358, "VISA resource name"=w362) -> ("error out"=w360:errorcluster, "VISA resource name out"=w359:refnum<visa-resource-name>)  [unwired: 5 in]
        n254 = call "Configure Measurement.vi"("Manual Range (1.0)"="Resistance Manual Range (1.0) 2", "error in (no error)"=w360, "Enable Auto Range (T:Enable)"="Enable Resistance Auto Range (T:Enable) 2", "Function (0: Volts)"=w357, "VISA resource name"=w359) -> ("error out"=w339:errorcluster, "VISA resource name out"=w340:refnum<visa-resource-name>)  [unwired: 5 in]
        n255 = local read "COMBO COMMAND"() -> (w338:string)
        n256 = call "Enable Output.vi"("error in (no error)"=w339, "Enable Output (T: Enable)"=TRUE, "VISA resource name"=w340) -> ("error out"=w343:errorcluster, "VISA resource name out"=w342:refnum<visa-resource-name>)  [unwired: 7 in]
        n257 = call-poly "Read.vi"("VISA resource name"=w342, "error in (no error)"=w343) -> ("Voltage"=→"Voltage 3":sgl, "Current"=w348:sgl, "Resistance"=→"Resistance 2":sgl)  [unwired: 7 in, 4 out]
        "Current 3" <- w348
        n258 = Search and Replace String(input string=w338, search string="keithleynew", replace string="1" ("replace string (\"\")")) -> (result string=w335:string)  [unwired: 5 in, 3 out]
        n259 = Multiply(x=w348, y=sgl 1000000.0) -> (x*y=→"Current Micro 2":sgl)
        n260 = case shown="\"False\", Default" w335 {
          tunnel: [FALSE TRUE] -> w333
          frame "False", Default {
            n261 = Wait (ms)(milliseconds to wait=u32 4000) -> ()  [unwired: 1 out]
          }
          frame "True" {
            n262 = Wait (ms)(milliseconds to wait=u32 4000) -> ()  [unwired: 1 out]
          }
        }
        n263 = local read "Quit"() -> (w332:bool)
        n264 = Or(x=w332, y=w333) -> (x .or. y?=w334:bool)
      }
    }
    frame #2 {
      # "Closing things down"
      n265 = VISA Close(VISA resource name=w655, error in (no error)=w656) -> (error out=w657:errorcluster)
      "LV TTi" <- w657
      n266 = VISA Close(VISA resource name=w653, error in (no error)=w652) -> ()  [unwired: 1 out]
      n267 = call <vilib>:"Simple Error Handler.vi"("error in (no error)"=w657) -> ()  [unwired: 4 in, 5 out]
      n268 = VISA Close(VISA resource name=w658, error in (no error)=w659) -> (error out=w660:errorcluster)
      "relay TTi" <- w660
      n269 = VISA Close(VISA resource name=w654, error in (no error)=w661) -> (error out=w662:errorcluster)
      "Chiller" <- w662
      n270 = call <vilib>:"Simple Error Handler.vi"("error in (no error)"=w660) -> ()  [unwired: 4 in, 5 out]
      n271 = call <vilib>:"Simple Error Handler.vi"("error in (no error)"=w662) -> ()  [unwired: 4 in, 5 out]
    }
  }
  n272 = property on="dewpoint" class="Str"("Text.FontSize"=u32 30 ("Text.Font:Size")) -> ()  [unwired: 2 in, 2 out]
